vi "template.vi"   [LabVIEW 2018]
uses:
  <vilib>/MediaMongrels Ltd/WebSockets/WebSockets/WebSocket Client/WebSocket Client.lvclass
  D:/software_setup/National Instruments/LabVIEW 2018/vi.lib/MediaMongrels Ltd/WebSockets/WebSockets/WebSocket/WebSocket.lvclass
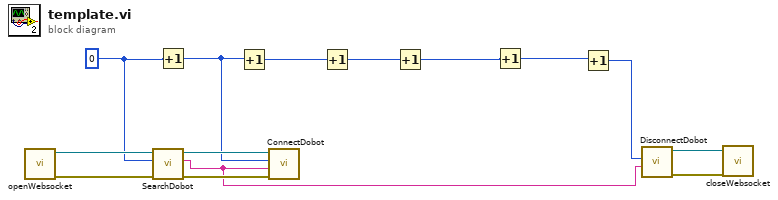
[diagram p0: block diagram]
diagram:
  w10 = 0 ("id")
  n1 = call <vilib>:"openWebsocket.vi"() -> ("error out"=w12:errorcluster, "WebSocket Client out"=w14:refnum<class "WebSocket Client.lvclass">)  [unwired: 10 in]
  n2 = call <vilib>:"SearchDobot.vi"("error in (no error)"=w12, "id"=w10, "WebSocket in"=w14) -> ("error out"=w11:errorcluster, "portName"=w3:string, "WebSocket out"=w13:refnum<class "WebSocket Client.lvclass">)  [unwired: 6 in]
  n3 = Increment(x=w10) -> (x+1=w9:i32)
  n4 = Increment(x=w9) -> (x+1=w7:i32)
  n5 = call <vilib>:"ConnectDobot.vi"("error in (no error)"=w11, "portName"=w3, "id"=w9, "WebSocket in"=w13) -> ()  [unwired: 5 in, 3 out]
  n6 = Increment(x=w7) -> (x+1=w6:i32)
  n7 = Increment(x=w6) -> (x+1=w5:i32)
  n8 = Increment(x=w5) -> (x+1=w4:i32)
  n9 = Increment(x=w4) -> (x+1=w8:i32)
  n10 = call <vilib>:"DisconnectDobot.vi"("portName"=w3, "id"=w8) -> ("error out"=w1:errorcluster, "WebSocket out"=w2:refnum<class "WebSocket.lvclass">)  [unwired: 7 in, 1 out]
  n11 = call <vilib>:"closeWebsocket.vi"("error in (no error)"=w1, "WebSocket in"=w2) -> ()  [unwired: 10 in]
